vi "Get Controls Mode.vi"(9 "Toggle Scoring Mode Requested?":bool, 10 "System is Idle?":bool, 11 "Operator Buttons":bool[](array[boolean])) -> (3 "Driver Controls Mode":T1)   [LabVIEW 2025]
uses:
  Driver Controls Mode.ctl
  <vilib>/Rock Robotics/WPI/Joystick/XBox Buttons Indexer.ctl
  194d4fd7-4f96-48c7-b586-d311dad63af0.vi
  fb9e03f0-c5c7-41f4-b181-bde3801f29a4.vi
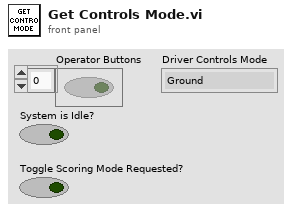
[diagram p1: front panel]
types:
  T1 = typedef "Driver Controls Mode.ctl" = enum16{"Ground", "Scoring"}
  T2 = typedef "XBox Buttons Indexer.ctl" = enum16{"A", "B", "X", "Y", "Left Bumper", "Right Bumper", "Back", "Start", "Left Joystick", "Right Joystick"}
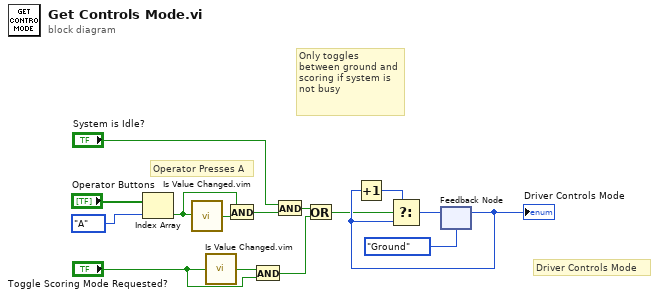
[diagram p0: block diagram]
diagram:
  # "Driver Controls Mode"
  # "Only toggles between ground and scoring if system is not busy"
  # "Operator Presses A"
  n1 = Index Array(array="Operator Buttons", index=XBox_Buttons_Indexer."A" ("XBox Buttons")) -> (element=w12:bool)
  n2 = call "Is Value Changed.vim"("value"=w12) -> ("changed or first call?"=w13:bool)
  n3 = call "Is Value Changed.vim"("value"="Toggle Scoring Mode Requested?") -> ("changed or first call?"=w3:bool)
  n4 = And(x=w12, y=w13) -> (x .and. y?=w6:bool)
  n5 = And(x=w3, y="Toggle Scoring Mode Requested?") -> (x .and. y?=w1:bool)
  n6 = And(x="System is Idle?", y=w6) -> (x .and. y?=w5:bool)
  n7 = Or(x=w5, y=w1) -> (x .or. y?=w4:bool)
  n8 = feedback #1(Driver_Controls_Mode."Ground") -> (w8:T1)
  "Driver Controls Mode" <- w8
  n9 = Increment(x=w8) -> (x+1=w9:T1)
  n10 = Select(t=w9, s=w4, f=w8) -> (s? t:f=w11:T1)
  n11 = feedback-in #1(w11) -> ()
